vi "test_AMI1700eth.vi"(10 "port":u16=7180, 11 "address":string="192.168.24.134") -> (0 "error out":errorcluster)   [LabVIEW 2019]
panel:
  out "status_init":bool
  out "status_N2_level":bool
  out "N2 level":dbl
  out "N":i32
  out "He level":dbl
  out "status_He_level":bool
  in  "stop":bool
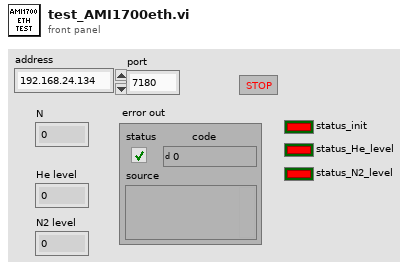
[diagram p1: front panel]
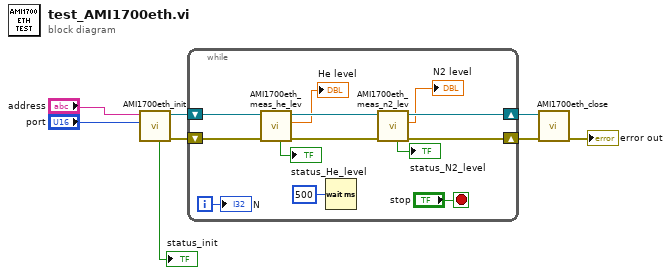
[diagram p0: block diagram]
diagram:
  n1 = call "AMI1700eth_init.vi"("port"="port", "address"="address") -> ("error out"=w5:errorcluster, "conn_id"=w6:refnum<k5>, "status"=→"status_init":bool)  [unwired: 7 in]
  n2 = while {
    shift-right: [w15] -> w2
    shift-left: w6 -> [w19]
    shift-right: [w13] -> w4
    shift-left: w5 -> [w18]
    i -> [w17]
    stop <- "stop" stop-if-true
    n3 = call "AMI1700eth_meas_he_lev.vi"("error in"=w18, "conn_id_in"=w19) -> ("error out"=w14:errorcluster, "level"=→"He level":dbl, "conn_id_out"=w16:refnum<k5>, "status"=→"status_He_level":bool)  [unwired: 6 in]
    n4 = Wait (ms)(milliseconds to wait=u32 500) -> ()  [unwired: 1 out]
    n5 = call "AMI1700eth_meas_n2_lev.vi"("error in"=w14, "conn_id_in"=w16) -> ("error out"=w13:errorcluster, "level"=→"N2 level":dbl, "conn_id_out"=w15:refnum<k5>, "status"=→"status_N2_level":bool)  [unwired: 6 in]
    "N" <- w17
  }
  n6 = call "AMI1700eth_close.vi"("error in"=w4, "conn_id"=w2) -> ("error out"=→"error out":errorcluster)  [unwired: 8 in, 1 out]
